vi "Swap DDS with CS.vi"(6 "Variant in":variant, 7 "Shift Pressed?":bool, 8 "error in (no error)":errorcluster, 10 "QD Combo Box Ref":refnum<vi>, 11 "QD Launch VI Ref":refnum<vi>) -> (0 "error out":errorcluster, 4 "Variant out":variant)   [LabVIEW 2017]
doc: "PLUGIN_DESCRIPTION: Replaces selected Diagram Disable Structure with Case Structure. Based on SAPHIR_DisableCode.vi.\nPLUGIN_DEFAULT_SHORTCUT:"
uses:
  <userlib>/_LAVACR/Scripting Tools/Scripting Tools.lvlib
panel:
  in  "Undo Name":string="DisableCode"
  # "More informations on : https://decibel.ni.com/content/groups/saphir-toolkit"
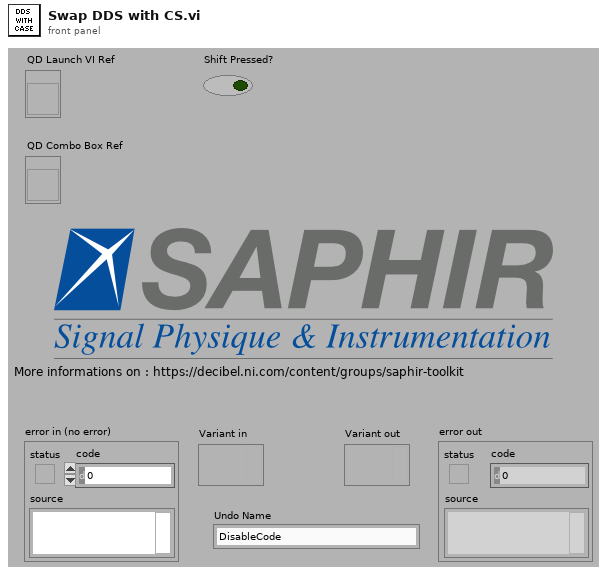
[diagram p1: front panel]
types:
  T1 = enum16{"Case Structure", "Stacked Sequence", "Event Structure", "Diagram Disable", "Conditional Disable", "While Loop", "For Loop", "Inplace Structure"}
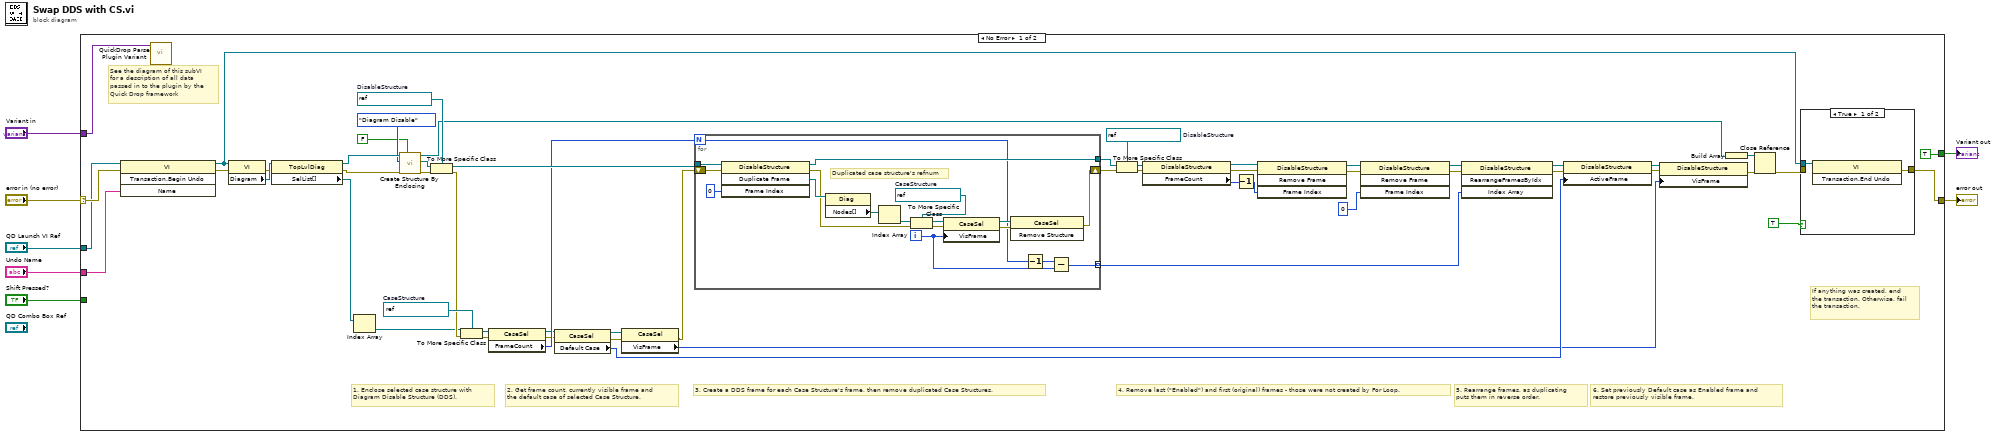
[diagram p0: block diagram]
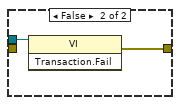
[diagram p2: hidden frame]
diagram:
  n1 = case shown="No Error" "error in (no error)" {
    selector: "error in (no error)" -> [w54 w86]
    tunnel: [w51 w86] -> w6
    tunnel: "QD Launch VI Ref" -> [w53 _]
    tunnel: "Variant in" -> [w55 _]
    tunnel: "Undo Name" -> [w52 _]
    tunnel: [TRUE _] -> w2
    tunnel: "Shift Pressed?" -> [_ _]
    frame No Error {
      w29 = refnum<vi> refnum  # DisableStructure
      w40 = refnum<vi> refnum  # CaseStructure
      w44 = refnum<vi> refnum  # DisableStructure
      # "6. Set previously Default case as Enabled frame and \nrestore previously visible frame."
      # "5. Rearrange frames, as duplicating \nputs them in reverse order."
      # "4. Remove last (\"Enabled\") and first (original) frames - those were not created by For Loop."
      # "3. Create a DDS frame for each Case Structure's frame, then remove duplicated Case Structures."
      # "2. Get frame count, currently visible frame and\nthe default case of selected Case Structure."
      # "1. Enclose selected case structure with\nDiagram Disable Structure (DDS)."
      # "If anything was created, end the transaction. Otherwise, fail the transaction."
      # "See the diagram of this subVI for a description of all data passed in to the plugin by the Quick Drop framework"
      n2 = invoke class="VI" method="Transaction.Begin Undo"(reference=w53, error in=w54, "Name"=w52) -> (reference out=w59:refnum<vi>, error out=w62:errorcluster)  [unwired: 1 in, 2 out]
      n3 = call <vilib>:"QuickDrop Parse Plugin Variant.vi"("QDKS Variant in"=w55) -> ()  [unwired: 12 in, 3 out]
      n4 = property class="VI"(reference=w59, error in=w62) -> (error out=w56:errorcluster, "Diagram"=w57:refnum<vi>)  [unwired: 1 out]
      n5 = property class="TopLvlDiag"(reference=w57, error in=w56) -> (reference out=w58:refnum<vi>, error out=w61:errorcluster, "SelList[]"=w49:refnum<vi>[])
      n6 = Index Array(array=w49) -> (element=w8:refnum<vi>)  [unwired: 1 in]
      n7 = call <userlib>:"Create Structure By Enclosing.vi"("Select everything except terminals ?"=FALSE, "error in (no error)"=w61, "Structure Type"=T1."Diagram Disable", "Diagram In"=w58) -> ("error out"=w45:errorcluster, "Structure Out"=w46:refnum<vi>, "Diagram Out"=w9:refnum<vi>)  [unwired: 5 in]
      n8 = To More Specific Class(target class=w44, reference=w46, error in=w45) -> (specific class reference=w42:refnum<vi>, error out=w31:errorcluster)
      n9 = To More Specific Class(target class=w40, reference=w8, error in=w31) -> (specific class reference=w39:refnum<vi>, error out=w32:errorcluster)
      n10 = property class="CaseSel"(reference=w39, error in=w32) -> (reference out=w37:refnum<vi>, error out=w36:errorcluster, "FrameCount"=w38:i32)
      n11 = property class="CaseSel"(reference=w37, error in=w36) -> (reference out=w34:refnum<vi>, error out=w33:errorcluster, "Default Case"=w35:i32)
      n12 = property class="CaseSel"(reference=w34, error in=w33) -> (error out=w10:errorcluster, "VisFrame"=w16:u32)  [unwired: 1 out]
      n13 = for {
        N: w38 -> [w67]
        tunnel: [w70] -> w28
        tunnel: w42 -> [w81]
        shift-right: [w71] -> w27
        shift-left: w10 -> [w80]
        tunnel: [w64] -> w15 mode=indexing
        i -> [w66]
        w76 = refnum<vi> refnum  # CaseStructure
        # "Duplicated case structure's refnum"
        n14 = invoke class="DisableStructure" method="Duplicate Frame"(reference=w81, error in=w80, "Frame Index"=u32 0) -> (reference out=w70:refnum<vi>, error out=w69:errorcluster, "Duplicate Frame"=w79:refnum<vi>)  [unwired: 1 in, 1 out]
        n15 = property class="Diag"(reference=w79) -> ("Nodes[]"=w78:refnum<vi>[])  [unwired: 1 in, 2 out]
        n16 = Index Array(array=w78) -> (element=w77:refnum<vi>)  [unwired: 1 in]
        n17 = To More Specific Class(target class=w76, reference=w77, error in=w69) -> (specific class reference=w75:refnum<vi>, error out=w74:errorcluster)
        n18 = property class="CaseSel"(reference=w75, error in=w74, "VisFrame"=w66) -> (reference out=w73:refnum<vi>, error out=w72:errorcluster)
        n19 = invoke class="CaseSel" method="Remove Structure"(reference=w73, error in=w72) -> (error out=w71:errorcluster)  [unwired: 1 in, 2 out]
        n20 = Decrement(x=w67) -> (x-1=w65:i32)
        n21 = Subtract(x=w65, y=w66) -> (x-y=w64:i32)
      }
      n22 = To More Specific Class(target class=w29, reference=w28, error in=w27) -> (specific class reference=w25:refnum<vi>, error out=w30:errorcluster)
      n23 = property class="DisableStructure"(reference=w25, error in=w30) -> (reference out=w24:refnum<vi>, error out=w26:errorcluster, "FrameCount"=w23:i32)
      n24 = Decrement(x=w23) -> (x-1=w20:i32)
      n25 = invoke class="DisableStructure" method="Remove Frame"(reference=w24, error in=w26, "Frame Index"=w20) -> (reference out=w22:refnum<vi>, error out=w21:errorcluster)  [unwired: 1 in, 2 out]
      n26 = invoke class="DisableStructure" method="Remove Frame"(reference=w22, error in=w21, "Frame Index"=u32 0) -> (reference out=w14:refnum<vi>, error out=w12:errorcluster)  [unwired: 1 in, 2 out]
      n27 = invoke class="DisableStructure" method="RearrangeFramesByIdx"(reference=w14, error in=w12, "Index Array"=w15) -> (reference out=w13:refnum<vi>, error out=w11:errorcluster)  [unwired: 1 in, 2 out]
      n28 = property class="DisableStructure"(reference=w13, error in=w11, "ActiveFrame"=w35) -> (reference out=w17:refnum<vi>, error out=w18:errorcluster)
      n29 = property class="DisableStructure"(reference=w17, error in=w18, "VisFrame"=w16) -> (error out=w43:errorcluster)  [unwired: 1 out]
      n30 = Build Array(w9) -> (w41:refnum<vi>[])
      n31 = Close Reference(reference=w41, error in (no error)=w43) -> (error out=w60:errorcluster)
      n32 = case shown="True" TRUE ("x") {
        tunnel: w59 -> [w82 w84]
        tunnel: [w83 w85] -> w51
        tunnel: w60 -> [_ _]
        frame True {
          n33 = invoke class="VI" method="Transaction.End Undo"(reference=w82) -> (error out=w83:errorcluster)  [unwired: 2 in, 2 out]
        }
        frame False {
          n34 = invoke class="VI" method="Transaction.Fail"(reference=w84) -> (error out=w85:errorcluster)  [unwired: 2 in, 2 out]
        }
      }
    }
    frame Error {
    }
  }
  "error out" <- w6
  "Variant out" <- w2
